vi "DAQDIGITAL.vi"() -> ()   [LabVIEW 2020, in "Acquisition.lvlib"]
uses:
  Acquisition.lvlib
  <vilib>/DAQmx/read.llb/DAQmx Read (Digital 1D Bool NChan 1Samp 1Line).vi
  <vilib>/DAQmx/read.llb/DAQmx Read (Digital 1D U32 NChan 1Samp).vi
  <vilib>/DAQmx/miscellaneous.llb/DAQmx Fill In Error Info.vi
panel:
  out "Boolean array 2":bool[](array[boolean])
  in  "DAQ LINEAS":tag
  in  "CANALES":tag[](array[tag])
  in  "error in 2":errorcluster caption="error in"
  in  "device name":tag
  in  "Canales":tag[](array[tag])
  out "Boolean array":bool[](array[boolean])
  out "Waveform Chart":u32[](graph)
  in  "stop":bool
  out "error out":errorcluster
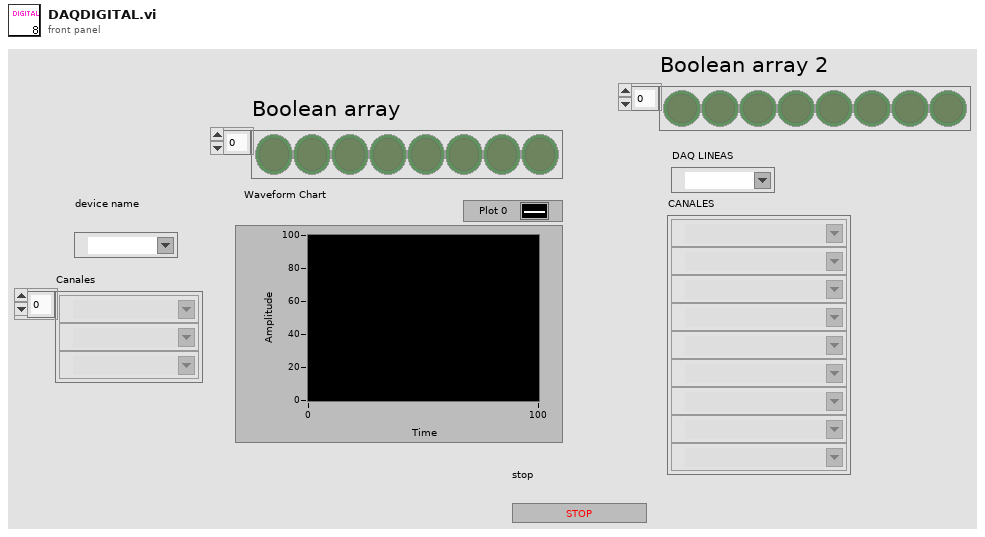
[diagram p1: front panel]
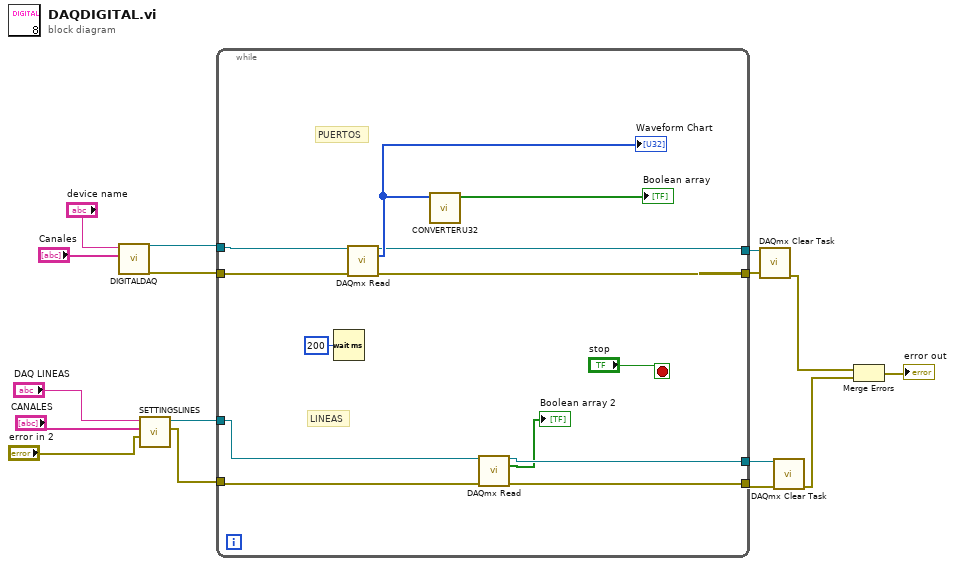
[diagram p0: block diagram]
diagram:
  n1 = call "DIGITALDAQ.vi"("Canales"="Canales", "DAQ Board Name"="device name") -> ("error out"=w12:errorcluster, "task out"=w11:refnum<k21>)  [unwired: 8 in]
  n2 = call "SETTINGSLINES.vi"("error in"="error in 2", "Canales"="CANALES", "DAQ Board Name"="DAQ LINEAS") -> ("error out"=w6:errorcluster, "task out"=w7:refnum<k21>)  [unwired: 7 in]
  n3 = while {
    tunnel: [w25] -> w16
    tunnel: [w24] -> w15
    tunnel: w12 -> [w23]
    tunnel: w11 -> [w22]
    tunnel: w7 -> [w21]
    tunnel: w6 -> [w20]
    tunnel: [w19] -> w5
    tunnel: [w18] -> w4
    stop <- "stop" stop-if-true
    # "LINEAS"
    # "PUERTOS"
    n4 = Wait (ms)(milliseconds to wait=u32 200) -> ()  [unwired: 1 out]
    n5 = call-poly <vilib>:"DAQmx Read.vi"("task/channels in"=w22, "error in"=w23) -> ("task out"=w25:refnum<k21>, "data"=w26:u32[], "error out"=w24:errorcluster)  [unwired: 11 in]
    "Waveform Chart" <- w26
    n6 = call "CONVERTERU32.vi"("data"=w26) -> ("Boolean array"=→"Boolean array":bool[])  [unwired: 10 in]
    n7 = call-poly <vilib>:"DAQmx Read.vi"("task/channels in"=w21, "error in"=w20) -> ("task out"=w19:refnum<k21>, "data"=→"Boolean array 2":bool[], "error out"=w18:errorcluster)  [unwired: 11 in]
  }
  n8 = call <vilib>:"DAQmx Clear Task.vi"("task in"=w16, "error in"=w15) -> ("error out"=w3:errorcluster)  [unwired: 13 in]
  n9 = call <vilib>:"DAQmx Clear Task.vi"("task in"=w5, "error in"=w4) -> ("error out"=w2:errorcluster)  [unwired: 13 in]
  n10 = Merge Errors(w3, w2) -> (→"error out":errorcluster)
